vi "温度.vi"(9 "U":dbl, 10 "Vcc":dbl, 11 "R":dbl) -> (1 "Rt":dbl, 2 "t":dbl)   [LabVIEW 2020]
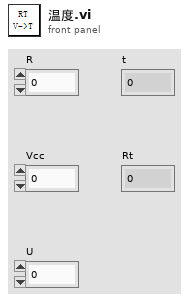
[diagram p1: front panel]
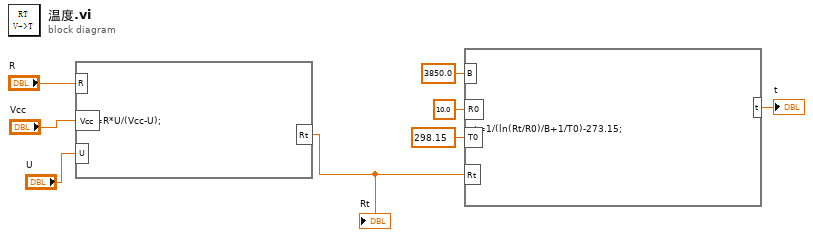
[diagram p0: block diagram]
diagram:
  n1 = formula code="Rt=R*U/(Vcc-U);"("R"="R", "Vcc"="Vcc", "U"="U") -> ("Rt"=w7:dbl)
  "Rt" <- w7
  n2 = formula code="t=1/(ln(Rt/R0)/B+1/T0)-273.15;"("B"=3850.0 ("输入变量"), "R0"=10.0 ("输入变量"), "T0"=298.15 ("输入变量"), "Rt"=w7) -> ("t"=→"t":dbl)
